vi "Read PizzaParams.vi"(8 "error in (no error)":errorcluster, 11 "Pizza":refnum<class "Pizza.lvclass">) -> (0 "error out":errorcluster, 2 "PizzaParams":T1, 3 "Pizza":refnum<class "Pizza.lvclass">)   [LabVIEW 2020, in "FactoryMethod.lvlib" / "PizzaFactoryMethod.lvlib" / "Pizza.lvclass"]
uses:
  Pizza.lvclass
  TypeDef/PizzaParams.ctl
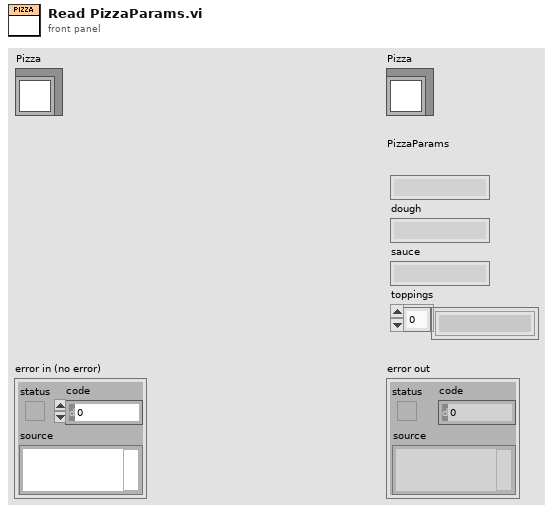
[diagram p1: front panel]
types:
  T1 = typedef "FactoryMethod.lvlib/PizzaFactoryMethod.lvlib/Pizza.lvclass/PizzaParams.ctl" = cluster{"name":string, "dough":string, "sauce":string, "toppings":string[]}
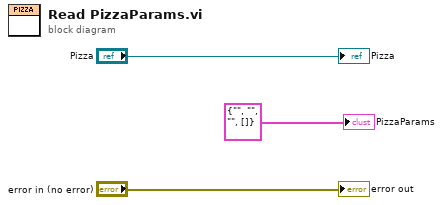
[diagram p0: block diagram]
diagram:
  "error out" <- "error in (no error)"
  "Pizza" <- "Pizza"
  "PizzaParams" <- T1 {"name"="", "dough"="", "sauce"="", "toppings"=[]} ("<ClassName>Params")
